vi "Ex7 Blurring Filters.vi"() -> ()   [LabVIEW 2020]
panel:
  in  "Noise Filter":u16(ring)=2 items=["Median Filter", "Gaussian Filter"]
  in  "Filter size Y (Filters 1)":i32=3
  in  "Filter size X (Filters 1)":i32=3
  in  "Kernel (Filters 1)":sgl[][](array[numeric])=[[1.0, 2.0, 1.0], [2.0, 4.0, 2.0], [1.0, 2.0, 1.0]]
  out "error out":errorcluster
  out "Filtered Image":T1(plugin-control)
  out "Image":T1(plugin-control)
  in  "Red or Hue Range (Color Threshold 1)":cluster{"Lower value":i32, "Upper value":i32}={"Lower value"=28, "Upper value"=90}
  in  "Green or Sat Range (Color Threshold 1)":cluster{"Lower value":i32, "Upper value":i32}={"Lower value"=0, "Upper value"=255}
  in  "Blue or Val  (Color Threshold 1)":cluster{"Lower value":i32, "Upper value":i32}={"Lower value"=5, "Upper value"=255}
  in  "Color Mode (Color Threshold 1)":u16(ring)=2 items=["RGB", "HSL", "HSV", "HSI"]
  in  "File Path":path
  # "EX.7 BLURRING FILTERS"
  # "Median Filter Inputs"
  # "Gaussian Filter Inputs"
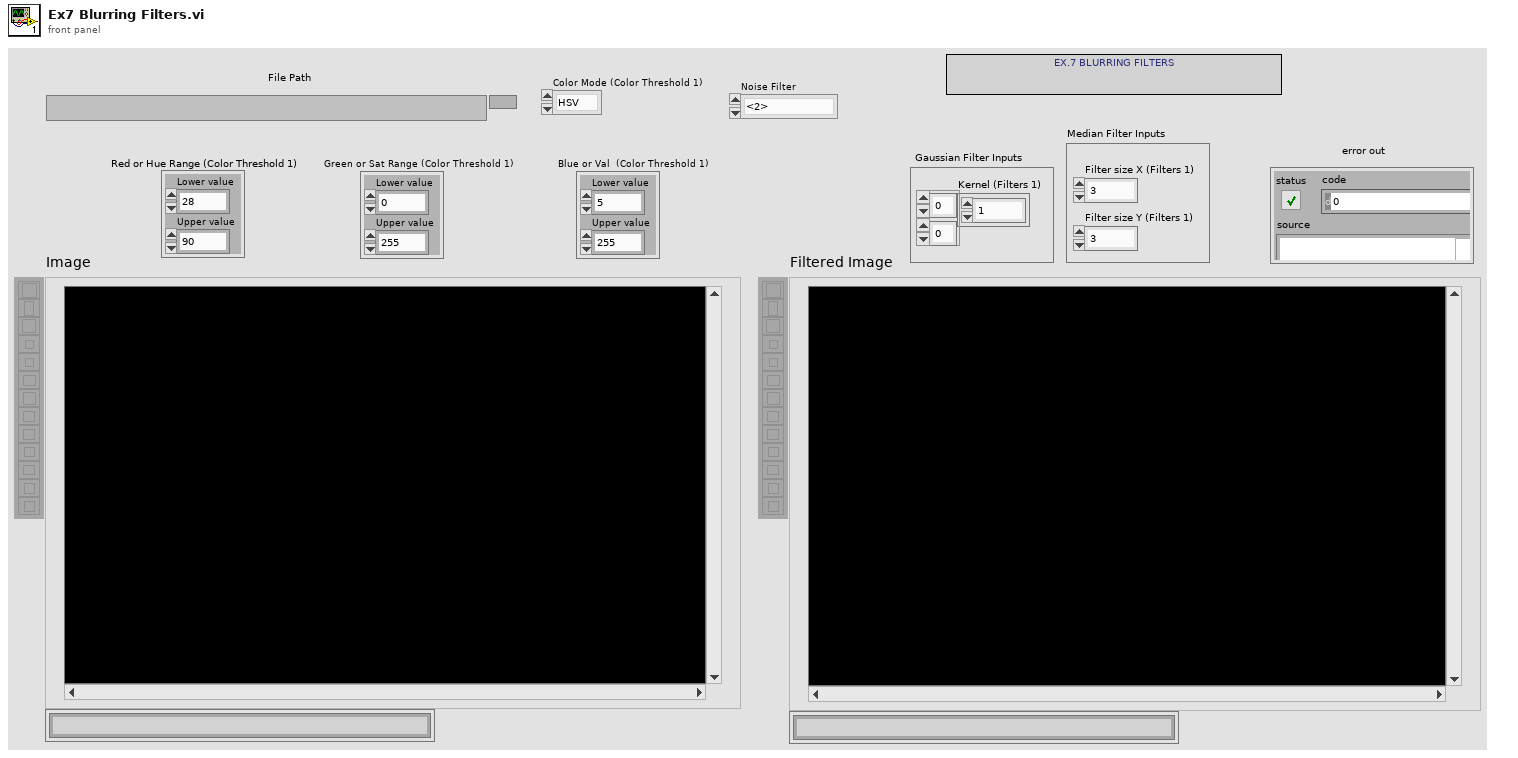
[diagram p1: front panel]
types:
  T1 = typedef "IMAQ Image.ctl" = refnum<image>
  T2 = typedef "Image Type" = u32
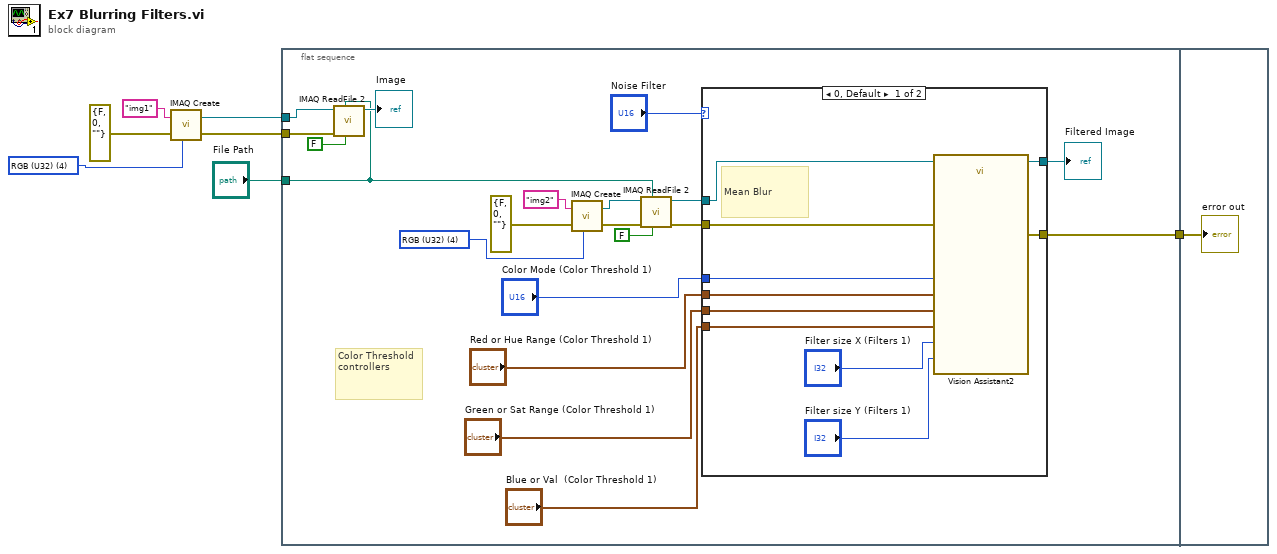
[diagram p0: block diagram]
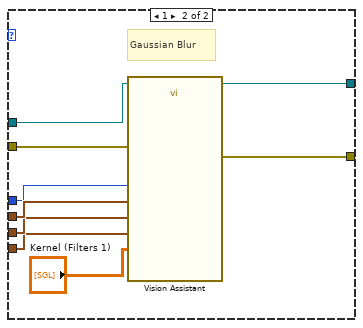
[diagram p2: hidden frame]
diagram:
  w1 = T2 4 items=["Grayscale (U8)", "Grayscale (I16)", "Grayscale (SGL)", "Complex (CSG)", "RGB (U32)", "HSL (U32)", "RGB (U64)", "Grayscale (U16)"] ("Image Type")
  n1 = call "IMAQ Create"("Image Name"="img1", "Image Type"=w1, "error in (no error)"=errorcluster {"status"=FALSE, "code"=0, "source"=""}) -> ("New Image"=w2:T1, "error out"=w3:errorcluster)  [unwired: 2 in]
  n2 = flat-sequence {
    tunnel: "File Path" -> [w16]
    tunnel: w3 -> [w26]
    tunnel: w2 -> [w25]
    tunnel: [w23] -> w7
    tunnel: w7 -> [w47]
    frame #0 {
      w20 = T2 4 items=["Grayscale (U8)", "Grayscale (I16)", "Grayscale (SGL)", "Complex (CSG)", "RGB (U32)", "HSL (U32)", "RGB (U64)", "Grayscale (U16)"] ("Image Type")
      # "Color Threshold controllers"
      n3 = call "IMAQ ReadFile 2"("Use File Path Image Type"=FALSE, "File Path"=w16, "error in (no error)"=w26, "Image"=w25) -> ("Image Out"=→"Image":T1)  [unwired: 3 in, 4 out]
      n4 = call "IMAQ Create"("Image Name"="img2", "Image Type"=w20, "error in (no error)"=errorcluster {"status"=FALSE, "code"=0, "source"=""}) -> ("New Image"=w19:T1, "error out"=w18:errorcluster)  [unwired: 2 in]
      n5 = call "IMAQ ReadFile 2"("Use File Path Image Type"=FALSE, "File Path"=w16, "error in (no error)"=w18, "Image"=w19) -> ("error out"=w14:errorcluster, "Image Out"=w15:T1)  [unwired: 3 in, 3 out]
      n6 = case shown="0, Default" "Noise Filter" {
        tunnel: [w32 w46] -> w23
        tunnel: w15 -> [w30 w45]
        tunnel: w14 -> [w31 w44]
        tunnel: "Red or Hue Range (Color Threshold 1)" -> [w36 w43]
        tunnel: "Green or Sat Range (Color Threshold 1)" -> [w35 w42]
        tunnel: [w33 w41] -> w11
        tunnel: "Blue or Val  (Color Threshold 1)" -> [w34 w40]
        tunnel: "Color Mode (Color Threshold 1)" -> [w37 w39]
        frame 0, Default {
          # "Mean Blur"
          n7 = call "Vision Assistant2"("Image In"=w30, "Color Mode (Color Threshold 1)"=w37, "Red or Hue Range (Color Threshold 1)"=w36, "Green or Sat Range (Color Threshold 1)"=w35, "Blue or Luma or Val or Inten Range (Color Threshold 1)"=w34, "Filter size X (Filters 1)"="Filter size X (Filters 1)", "error in"=w31, "Filter size Y (Filters 1)"="Filter size Y (Filters 1)") -> ("Image Out"=w33:T1, "error out"=w32:errorcluster)  [unwired: 18 in]
        }
        frame 1 {
          # "Gaussian Blur"
          n8 = call "Vision Assistant"("Image In"=w45, "Color Mode (Color Threshold 1)"=w39, "Red or Hue Range (Color Threshold 1)"=w43, "Green or Sat Range (Color Threshold 1)"=w42, "Blue or Luma or Val or Inten Range (Color Threshold 1)"=w40, "Kernel (Filters 1)"="Kernel (Filters 1)", "error in"=w44) -> ("Image Out"=w41:T1, "error out"=w46:errorcluster)  [unwired: 19 in]
        }
      }
      "Filtered Image" <- w11
    }
    frame #1 {
      "error out" <- w47
    }
  }
